vi "CAEN_HV_subvi_deinitialize.vi"(1 "Handle 2":dbl, 2 "Handle 1":dbl, 3 "error in":errorcluster) -> (0 "error out":errorcluster)   [LabVIEW 2012]
uses:
  CAEN/labview/CAENHVWrapper/CAENHVWrapper.lvlib
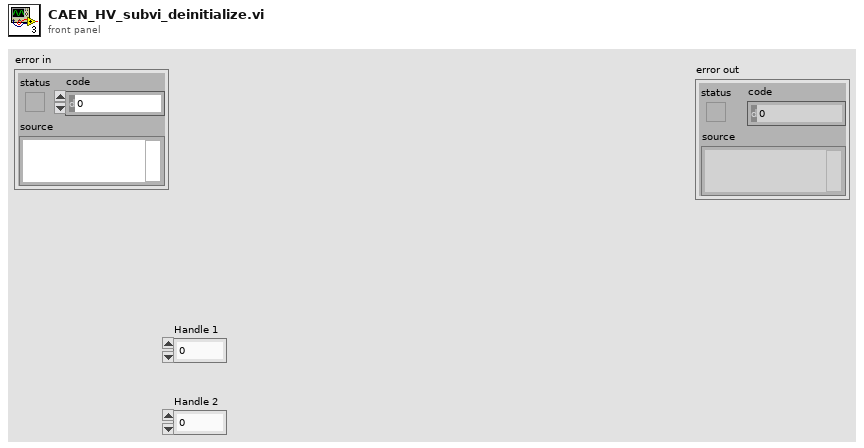
[diagram p1: front panel]
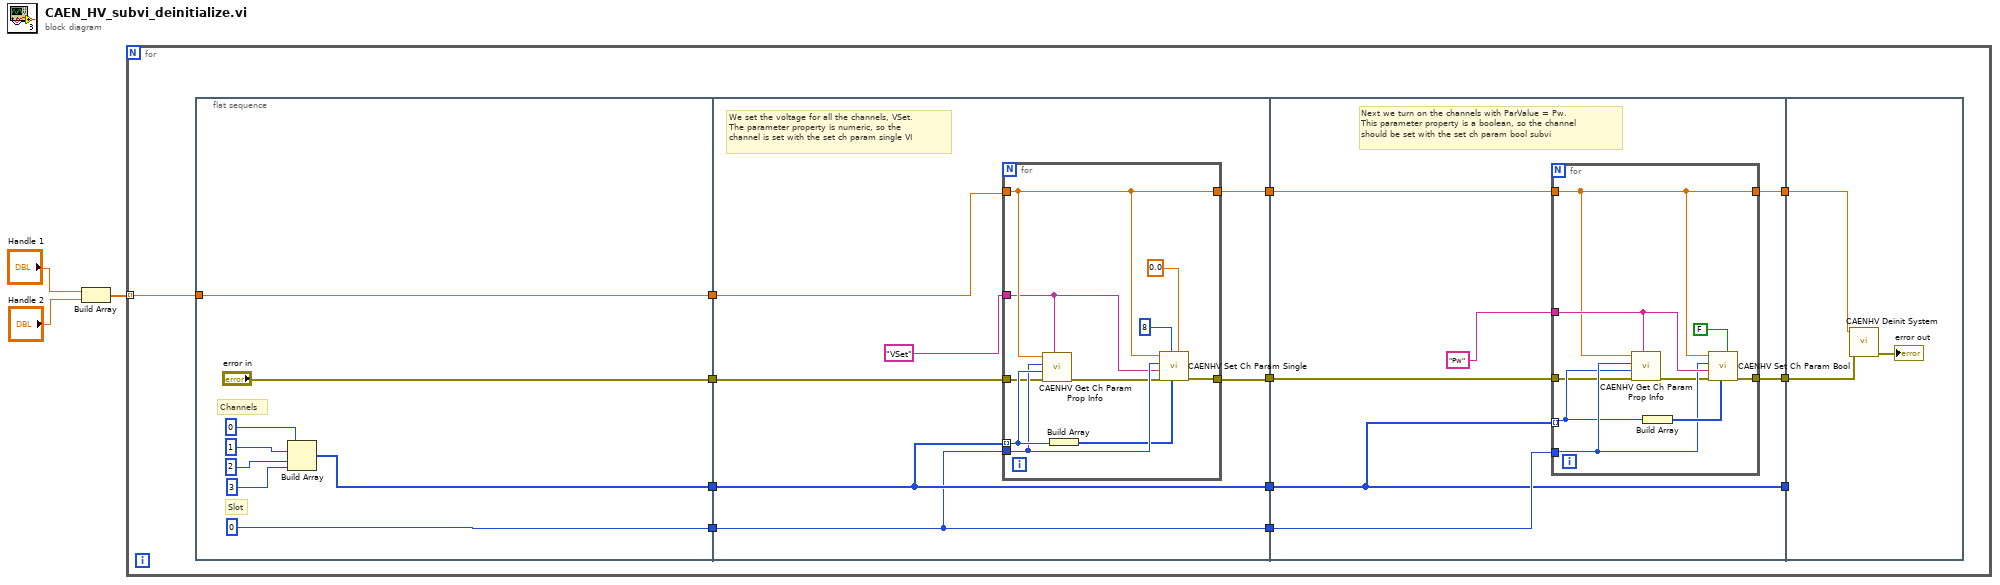
[diagram p0: block diagram]
diagram:
  n1 = Build Array("Handle 1", "Handle 2") -> (w1:dbl[])
  n2 = for {
    tunnel: w1 -> [w4] mode=indexing
    n3 = flat-sequence {
      tunnel: [w23] -> w15
      tunnel: [0] -> w14
      tunnel: ["error in"] -> w13
      tunnel: [w16] -> w5
      tunnel: w4 -> [w16]
      tunnel: [w30] -> w12
      tunnel: [w27] -> w11
      tunnel: [w29] -> w10
      tunnel: [w28] -> w9
      tunnel: w15 -> [w28]
      tunnel: w14 -> [w27]
      tunnel: w13 -> [w25]
      tunnel: w5 -> [w24]
      tunnel: w12 -> [w46]
      tunnel: w11 -> [w42]
      tunnel: w10 -> [w45]
      tunnel: w9 -> [w41]
      tunnel: [w44] -> w8
      tunnel: [w43] -> w7
      tunnel: [w41] -> w6
      tunnel: w8 -> [w58]
      tunnel: w7 -> [w57]
      tunnel: w6 -> [_]
      frame #0 {
        # "Slot"
        # "Channels"
        n4 = Build Array(0, 1, 2, 3) -> (w23:i32[])
      }
      frame #1 {
        # "We set the voltage for all the channels, VSet.\nThe parameter property is numeric, so the\nchannel is set with the set ch param single VI"
        n5 = for {
          tunnel: "VSet" ("Setvoltage") -> [w37]
          tunnel: w28 -> [w40] mode=indexing
          tunnel: w27 -> [w38]
          tunnel: w24 -> [w39]
          tunnel: [w39] -> w30
          tunnel: [w36] -> w29
          tunnel: w25 -> [w31]
          n6 = call "CAENHV Get Ch Param Prop Info.vi"("ParName"=w37, "error in (no error)"=w31, "Ch"=w40, "slot"=w38, "handle"=w39) -> ("error out"=w34:errorcluster)  [unwired: 4 in, 2 out]
          n7 = Build Array(w40) -> (w35:i32[])
          n8 = call "CAENHV Set Ch Param Single.vi"("ParValue"=sgl 0.0, "ChList"=w35, "ChNum (1)"=u16 8, "error in (no error)"=w34, "ParName"=w37, "slot"=w38, "handle"=w39) -> ("error out"=w36:errorcluster)  [unwired: 4 in]
        }
      }
      frame #2 {
        # "Next we turn on the channels with ParValue = Pw. \nThis parameter property is a boolean, so the channel\nshould be set with the set ch param bool subvi"
        n9 = for {
          tunnel: [w56] -> w43
          tunnel: "Pw" ("ParName") -> [w55]
          tunnel: w46 -> [w53]
          tunnel: [w53] -> w44
          tunnel: w42 -> [w52]
          tunnel: w41 -> [w51] mode=indexing
          tunnel: w45 -> [w50]
          n10 = call "CAENHV Get Ch Param Prop Info.vi"("ParName"=w55, "error in (no error)"=w50, "Ch"=w51, "slot"=w52, "handle"=w53) -> ("error out"=w49:errorcluster)  [unwired: 4 in, 2 out]
          n11 = Build Array(w51) -> (w54:i32[])
          n12 = call "CAENHV Set Ch Param Bool.vi"("ParValue"=FALSE, "ChList"=w54, "error in (no error)"=w49, "ParName"=w55, "slot"=w52, "handle"=w53) -> ("error out"=w56:errorcluster)  [unwired: 5 in]
        }
      }
      frame #3 {
        n13 = call "CAENHV Deinit System.vi"("error in (no error)"=w57, "handle"=w58) -> ("error out"=→"error out":errorcluster)  [unwired: 9 in]
      }
    }
  }
